vi "Chebfit.vi"(9 "degree":u16=2, 10 "Y":dbl[](array[numeric]), 11 "X":dbl[](array[numeric])) -> (3 "C":dbl[](array[numeric]) format="%.2f")   [LabVIEW 2025]
uses:
  <vilib>/Analysis/7linalg.llb/Solve Linear Equations (single right hand).vi
  <vilib>/Analysis/baseanly.llb/Solve Linear Equations By Cholesky.vi
  <vilib>/Analysis/baseanly.llb/Real Matrix to Compact Array.vi
  <vilib>/Analysis/baseanly.llb/Real Compact Tri-Matrix Linear Eqs.vi
  <vilib>/Analysis/7linalg.llb/Solve Linear Eqs (General).vi
  <vilib>/Analysis/7linalg.llb/Solve Linear Eqs (Gen, single right hand).vi
  <vilib>/Analysis/NI_AALPro.lvlib
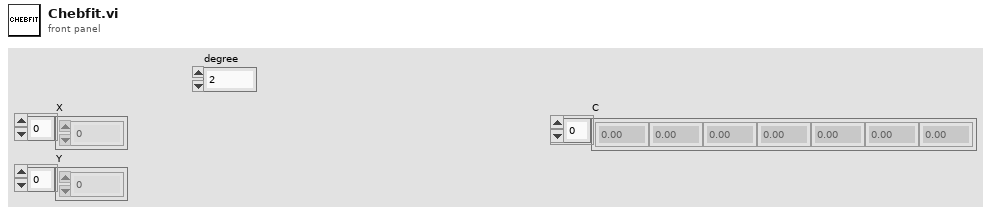
[diagram p1: front panel]
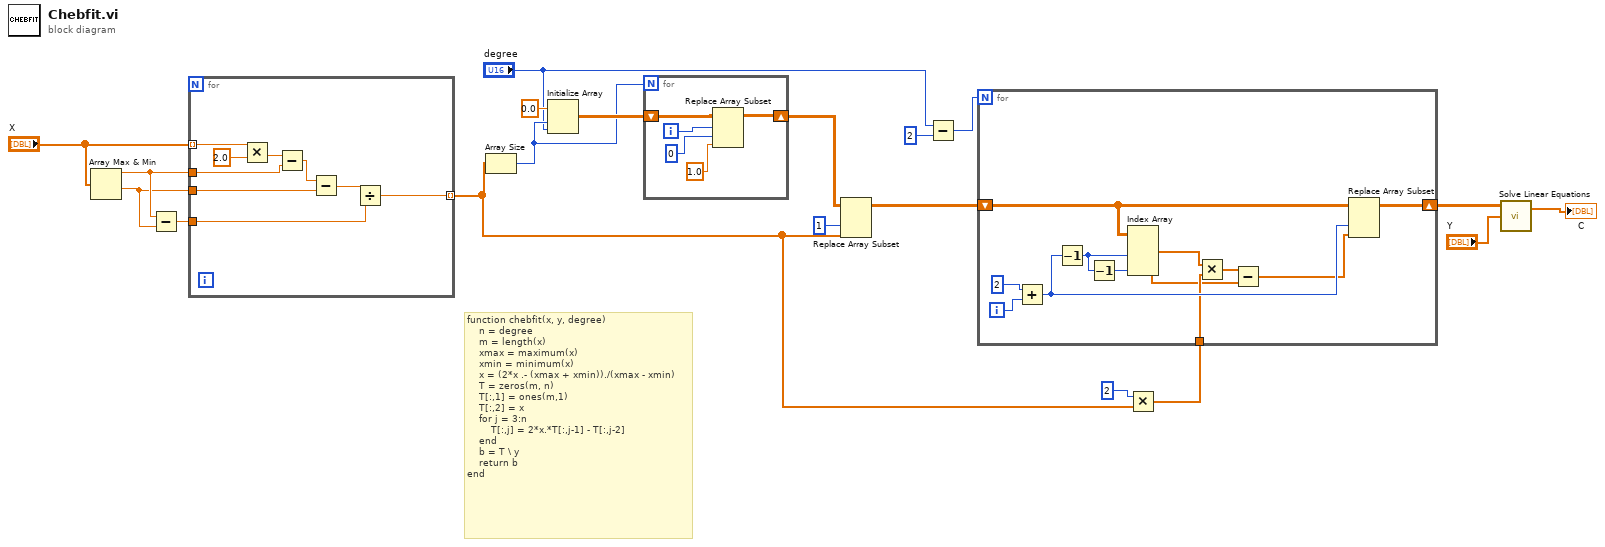
[diagram p0: block diagram]
diagram:
  # "function chebfit(x, y, degree)\n    n = degree\n    m = length(x)\n    xmax = maximum(x)\n    xmin = minimum(x)\n    x = (2*x .- (xmax + xmin))./(xmax - xmin)\n    T = zeros(m, n)\n    T[:,1] = ones(m,1)\n    T[:,2] = x\n    for j = 3:n\n        T[:,j] = 2*x.*T[:,j-1] - T[:,j-2]\n    end\n    b = T \\ y\n    return b\nend"
  n1 = Array Max & Min(array="X") -> (max value=w18:dbl, min value=w17:dbl)  [unwired: 2 out]
  n2 = Subtract(x=w18, y=w17) -> (x-y=w16:dbl)
  n3 = for {
    tunnel: "X" -> [w28] mode=indexing
    tunnel: w18 -> [w25]
    tunnel: w17 -> [w23]
    tunnel: w16 -> [w21]
    tunnel: [w20] -> w4 mode=indexing
    n4 = Multiply(x=w28, y=2.0) -> (x*y=w26:dbl)
    n5 = Subtract(x=w26, y=w25) -> (x-y=w24:dbl)
    n6 = Subtract(x=w24, y=w23) -> (x-y=w22:dbl)
    n7 = Divide(x=w22, y=w21) -> (x/y=w20:dbl)
  }
  n8 = Array Size(array=w4) -> (size(s)=w10:i32)
  n9 = Initialize Array(0.0 ("element"), w10, "degree") -> (w14:dbl[][])
  n10 = for {
    N: w10 -> [_]
    shift-right: [w31] -> w13
    shift-left: w14 -> [w33]
    i -> [w30]
    n11 = Replace Array Subset(array=w33, new element=1.0 ("new element/subarray"), index (row)=w30, index (col)=0 ("disabled index (col)")) -> (w31:dbl[][])
  }
  n12 = Replace Array Subset(array=w13, new element=w4, index (col)=1 ("index (row)")) -> (w11:dbl[][])  [unwired: 1 in]
  n13 = Subtract(x="degree", y=2) -> (x-y=w8:i32)
  n14 = Multiply(x=2, y=w4) -> (x*y=w6:dbl[])
  n15 = for {
    N: w8 -> [_]
    tunnel: w6 -> [w38]
    shift-right: [w34] -> w2
    shift-left: w11 -> [w43]
    i -> [w45]
    n16 = Add(x=2, y=w45) -> (x+y=w42:i32)
    n17 = Decrement(x=w42) -> (x-1=w41:i32)
    n18 = Decrement(x=w41) -> (x-1=w40:i32)
    n19 = Index Array(array=w43, index (col) #1=w41, index (col) #2=w40) -> (element #1=w39:dbl[], element #2=w36:dbl[])  [unwired: 2 in]
    n20 = Multiply(x=w39, y=w38) -> (x*y=w37:dbl[])
    n21 = Subtract(x=w37, y=w36) -> (x-y=w35:dbl[])
    n22 = Replace Array Subset(array=w43, new element=w35, index (col)=w42) -> (w34:dbl[][])  [unwired: 1 in]
  }
  n23 = call-poly <vilib>:"Solve Linear Equations.vi"("Known Vector"="Y", "Input Matrix"=w2) -> ("Solution Vector"=→"C":dbl[])  [unwired: 1 in, 1 out]
